vi "GetScanListLength.vi"(8 "Error In":errorcluster, 11 "Keithley 7001 In":refnum<visa-resource-name>) -> (0 "Error Out":errorcluster, 2 "Scan List Length":u16, 3 "Keithley 7001 Out":refnum<visa-resource-name>)   [LabVIEW 2012, in "Keithley-7001.lvlib"]
uses:
  Keithley-7001.lvlib
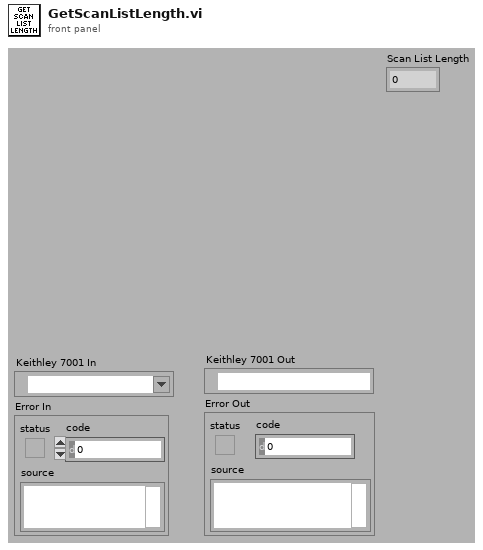
[diagram p1: front panel]
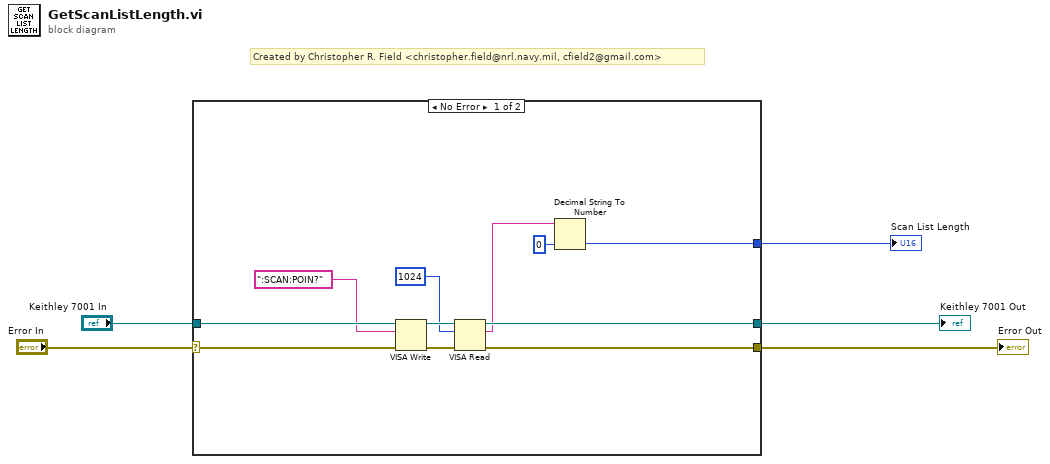
[diagram p0: block diagram]
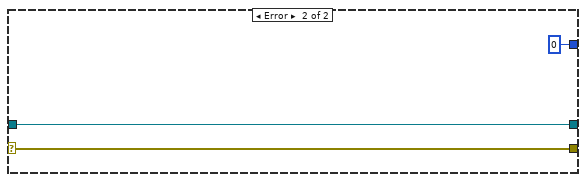
[diagram p2: hidden frame]
diagram:
  # "Created by Christopher R. Field <christopher.field@nrl.navy.mil, cfield2@gmail.com>"
  n1 = case shown="No Error" "Error In" {
    selector: "Error In" -> [w6 w19]
    tunnel: "Keithley 7001 In" -> [w14 w18]
    tunnel: [w13 w18] -> w4
    tunnel: [w12 w19] -> w3
    tunnel: [w8 u16 0] -> w2
    frame No Error {
      n2 = VISA Write(VISA resource name=w14, write buffer=":SCAN:POIN?", error in (no error)=w6) -> (VISA resource name out=w16:refnum<visa-resource-name>, error out=w15:errorcluster)  [unwired: 1 out]
      n3 = VISA Read(VISA resource name=w16, byte count=u32 1024, error in (no error)=w15) -> (VISA resource name out=w13:refnum<visa-resource-name>, read buffer=w9:string, error out=w12:errorcluster)  [unwired: 1 out]
      n4 = Decimal String To Number(string=w9, default (0L)=u16 0 ("default (0 I32)")) -> (number=w8:u16)  [unwired: 1 in, 1 out]
    }
    frame Error {
    }
  }
  "Keithley 7001 Out" <- w4
  "Error Out" <- w3
  "Scan List Length" <- w2
